vi "Redirect Assemblies in Veristand Steps Project XML.vi"() -> ()   [LabVIEW 2013, in "Assembly Redirection VIs.lvlib"]
uses:
  Assembly Redirection VIs.lvlib
  <vilib>/xml/NI_XML.lvlib
  <resource>/objmgr/DOMUserDefRef.rc
  <vilib>/xml/Load XML File.vi
  <vilib>/xml/Close Reference(Node).vi
  <vilib>/ni/Simple XML/Simple XML.lvlib
  <vilib>/xml/Close Reference(NNMap).vi
  <vilib>/NI/Simple XML/_polymorphics/Create Tag - Child with Text.vi
panel:
  in  "New VS Assembly Version":string="2016.0.0.0"
  in  "New VS Assembly Version (GAC)":string="4.0.2016.0.9.9"
  out "New Assembly Reference Include Strings":string[](array[string])=["NationalInstruments.TestStand.Interop.API, Version=1.2.3.4, Culture=neutral, PublicKeyToken=ad9244eb3b825cd8, processorArchitecture=MSIL", "NationalInstruments.TestStand.Interop.UI, Version=1.2.3.4, Culture=neutral, PublicKeyToken=ad9244eb3b825cd8, processorArchitecture=MSIL", "NationalInstruments.TestStand.Interop.UI.AxControls, Version=1.2.3.4, Culture=neutral, PublicKeyToken=ad9244eb3b825cd8, processorArchitecture=MSIL", "NationalInstruments.TestStand.Interop.UI.Support, Version=1.2.3.4, Culture=neutral, PublicKeyToken=ad9244eb3b825cd8, processorArchitecture=MSIL", "NationalInstruments.TestStand.Interop.Utility, Version=5.6.7.8, Culture=neutral, processorArchitecture=x86", "NationalInstruments.VeriStand, Version=2016.0.0.0, Culture=neutral, PublicKeyToken=a6d690c380daa308, processorArchitecture=MSIL", "NationalInstruments.VeriStand.ClientAPI, Version=2016.0.0.0, Culture=neutral, PublicKeyToken=a6d690c380daa308, processorArchitecture=MSIL", "NationalInstruments.VeriStand.DataTypes, Version=2016.0.0.0, Culture=neutral, PublicKeyToken=a6d690c380daa308, processorArchitecture=MSIL", "NationalInstruments.VeriStand.RealTimeSequenceDefinitionApi, Version=2016.0.0.0, Culture=neutral, PublicKeyToken=a6d690c380daa308, processorArchitecture=MSIL", "NationalInstruments.VeriStand.SystemDefinitionAPI, Version=2016.0.0.0, Culture=neutral, PublicKeyToken=a6d690c380daa308, processorArchitecture=MSIL", "NationalInstruments.VeriStand.SystemStorage, Version=2016.0.0.0, Culture=neutral, PublicKeyToken=a6d690c380daa308, processorArchitecture=MSIL", "NationalInstruments.VeriStand.SystemStorageUI, Version=2016.0.0.0, Culture=neutral, PublicKeyToken=a6d690c380daa308, processorArchitecture=MSIL", "NationalInstruments.VeriStand.WorkspaceMacro, Version=2016.0.0.0, Culture=neutral, PublicKeyToken=a6d690c380daa308, processorArchitecture=MSIL"]
  out "New Assembly HintPath Properties":string[](array[string])=["..\\..\\..\\..\\..\\..\\..\\..\\..\\Program Files (x86)\\National Instruments\\TestStand 2016\\API\\DotNet\\Assemblies\\CurrentVersion\\NationalInstruments.TestStand.Interop.API.dll", "..\\..\\..\\..\\..\\..\\..\\..\\..\\Program Files (x86)\\National Instruments\\TestStand 2016\\API\\DotNet\\Assemblies\\CurrentVersion\\NationalInstruments.TestStand.Interop.UI.dll", "..\\..\\..\\..\\..\\..\\..\\..\\..\\Program Files (x86)\\National Instruments\\TestStand 2016\\API\\DotNet\\Assemblies\\CurrentVersion\\NationalInstruments.TestStand.Interop.UI.AxControls.dll", "..\\..\\..\\..\\..\\..\\..\\..\\..\\Program Files (x86)\\National Instruments\\TestStand 2016\\API\\DotNet\\Assemblies\\CurrentVersion\\NationalInstruments.TestStand.Interop.UISupport.dll", "..\\..\\..\\..\\..\\..\\..\\..\\..\\Program Files (x86)\\National Instruments\\TestStand 2016\\Bin\\NationalInstruments.TestStand.Utility.dll", "..\\..\\..\\..\\..\\..\\..\\..\\Windows\\Microsoft.NET\\assembly\\GAC_MSIL\\NationalInstruments.VeriStand\\v4.0_2016.0.9.9__a6d690c380daa308\\NationalInstruments.VeriStand.dll", "..\\..\\..\\..\\..\\..\\..\\..\\Windows\\Microsoft.NET\\assembly\\GAC_MSIL\\NationalInstruments.VeriStand.ClientAPI\\v4.0_2016.0.9.9__a6d690c380daa308\\NationalInstruments.VeriStand.ClientAPI.dll", "..\\..\\..\\..\\..\\..\\..\\..\\Windows\\Microsoft.NET\\assembly\\GAC_MSIL\\NationalInstruments.VeriStand.DataTypes\\v4.0_2016.0.9.9__a6d690c380daa308\\NationalInstruments.VeriStand.DataTypes.dll", "..\\..\\..\\..\\..\\..\\..\\..\\Windows\\Microsoft.NET\\assembly\\GAC_MSIL\\NationalInstruments.VeriStand.RealTimeSequenceDefinitionAPI\\v4.0_2016.0.9.9__a6d690c380daa308\\NationalInstruments.VeriStand.RealTimeSequenceDefinitionAPI.dll", "..\\..\\..\\..\\..\\..\\..\\..\\Windows\\Microsoft.NET\\assembly\\GAC_MSIL\\NationalInstruments.VeriStand.SystemDefinitionAPI\\v4.0_2016.0.9.9__a6d690c380daa308\\NationalInstruments.VeriStand.SystemDefinition.dll", "..\\..\\..\\..\\..\\..\\..\\..\\Windows\\Microsoft.NET\\assembly\\GAC_MSIL\\NationalInstruments.VeriStand.SystemStorage\\v4.0_2016.0.9.9__a6d690c380daa308\\NationalInstruments.VeriStand.SystemStorage.dll", "..\\..\\..\\..\\..\\..\\..\\..\\Windows\\Microsoft.NET\\assembly\\GAC_MSIL\\NationalInstruments.VeriStand.SystemStorageUI\\v4.0_2016.0.9.9__a6d690c380daa308\\NationalInstruments.VeriStand.SystemStorageUI.dll", "..\\..\\..\\..\\..\\..\\..\\..\\Windows\\Microsoft.NET\\assembly\\GAC_MSIL\\NationalInstruments.VeriStand.WorkspaceMacro\\v4.0_2016.0.9.9__a6d690c380daa308\\NationalInstruments.VeriStand.WorkspaceMacro.dll"]
  in  "New TS Version":dbl=2016.0 format="%#_6f"
  out "error out":errorcluster
  in  "Path to New XML File":path=path "C:/Users/achurch/Documents/Source/XML Mutation Code/Examples XML Files/VeristandSteps_mod.csproj" caption="Path to New RemoveOldInsertionPaletteItems project file"
  in  "New TS Utility Assembly Version":string="5.6.7.8"
  in  "New TS Interop Assembly Version":string="1.2.3.4"
  in  "XML file path":path=path "C:/Users/achurch/Documents/Source/XML Mutation Code/Examples XML Files/VeristandSteps.csproj" caption="Path to Old RemoveOldInsertionPaletteItems project file"
  # "Arguments\n1: original path (string)\n2: new path (string)\n3: TS Version (2014)\n4: TS Interop Assembly Version (14.0.0.0)\n5: TS Utility Assembly Version (14.0.0.0)\n6: VS Assembly Version (GAC format, 4.0.2016.0.0.0)\n7: VS Assembly Version (2016.0.0.0)"
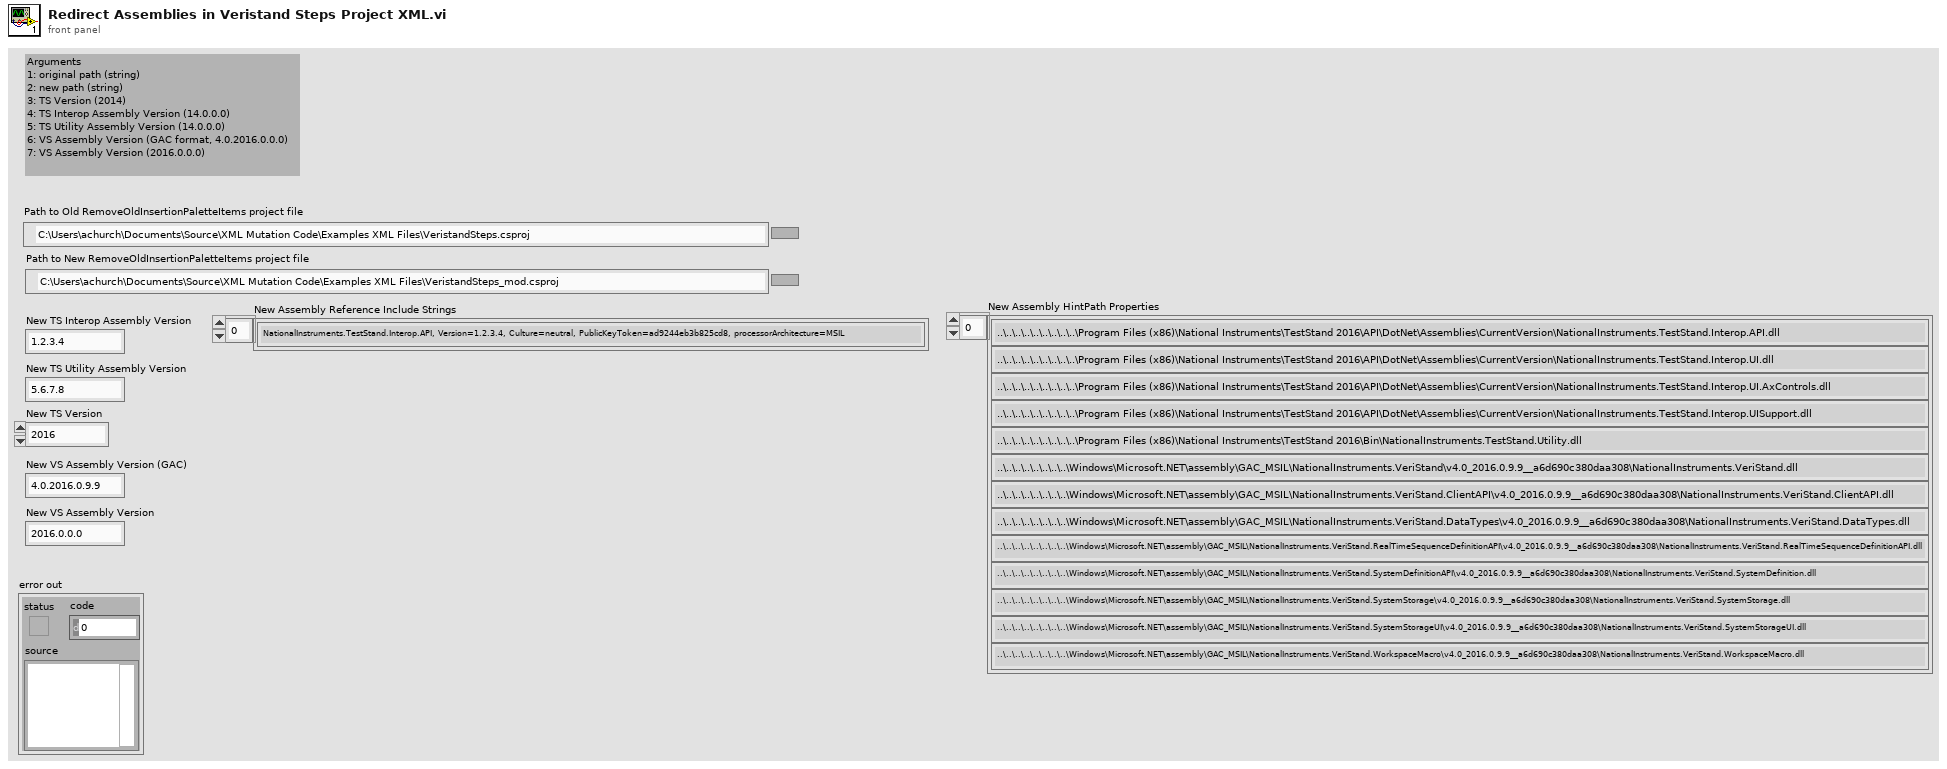
[diagram p1: front panel]
types:
  T1 = enum32{"invalid app kind", "Development System", "Run Time System", "Student Edition", "Embedded LabVIEW", "Evaluation", "Custom"}
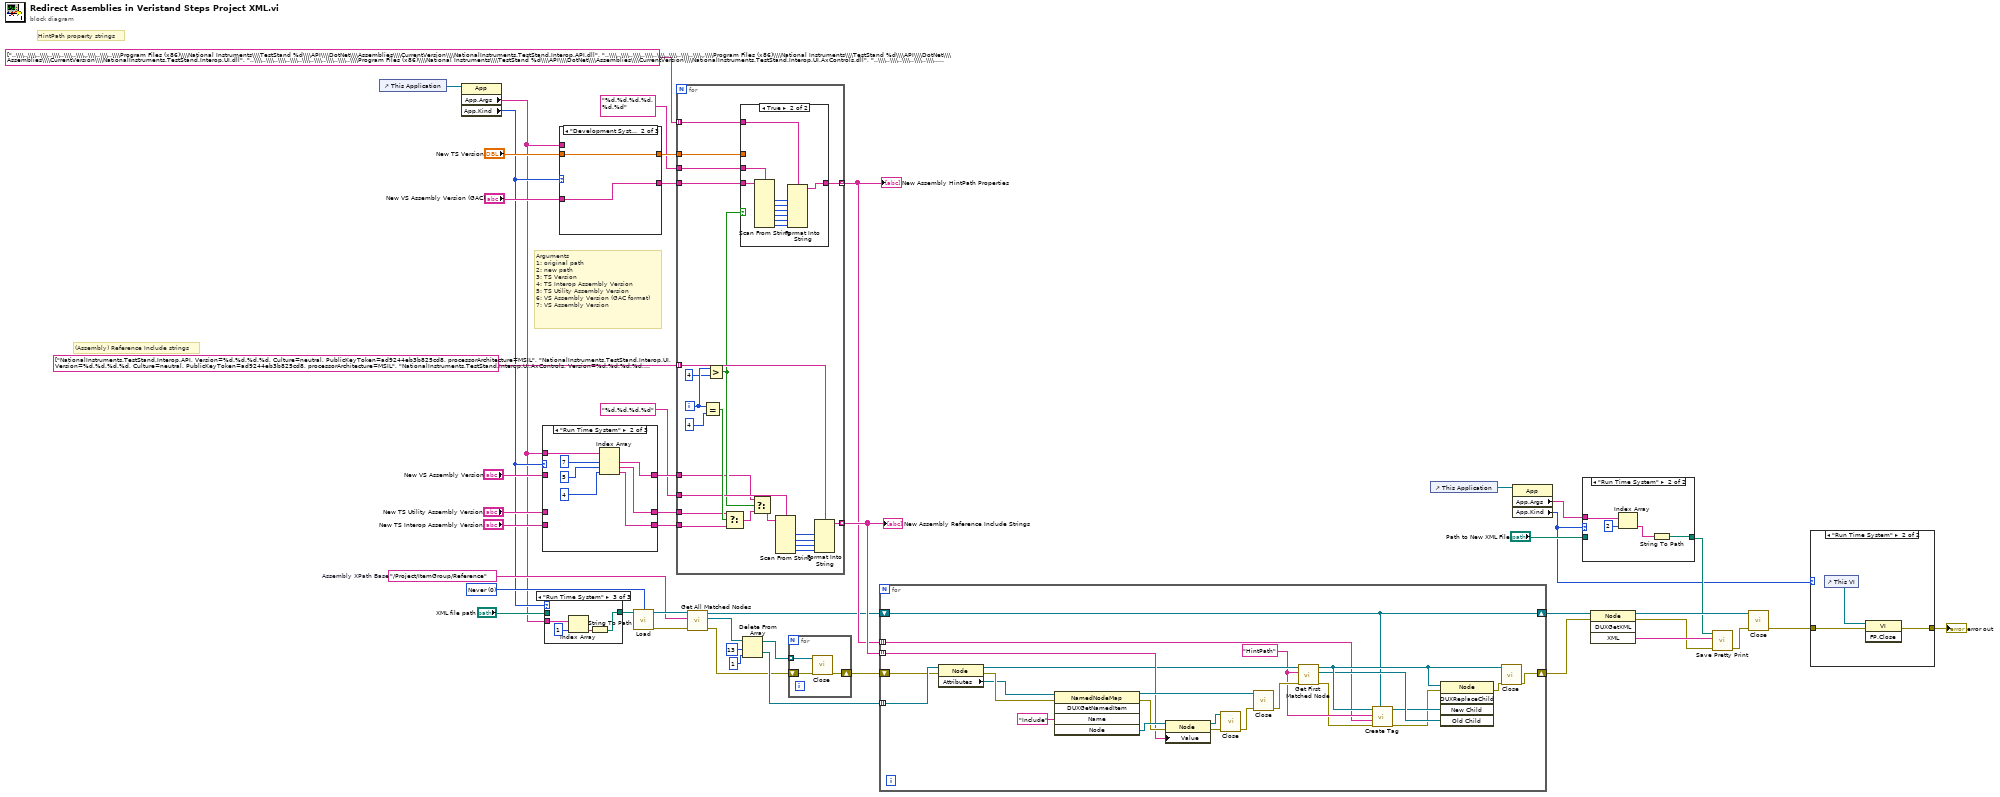
[diagram p0: block diagram]
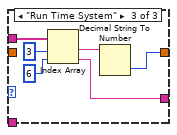
[diagram p9: hidden frame]
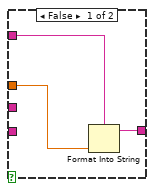
[diagram p10: hidden frame]
diagram:
  w43 = "/Project/ItemGroup/Reference"  # Assembly XPath Base
  w46 = 0 items=["Never", "Always", "Auto"] ("validate on load (Auto)")
  # "Arguments\n1: original path\n2: new path\n3: TS Version\n4: TS Interop Assembly Version\n5: TS Utility Assembly Version\n6: VS Assembly Version (GAC format)\n7: VS Assembly Version"
  # "(Assembly) Reference Include strings"
  # "HintPath property strings"
  n1 = control-ref of="This Application"() -> (w24:refnum<vi>)
  n2 = property class="App"(reference=w24) -> ("App.Args"=w8:string[], "App.Kind"=w11:T1)  [unwired: 1 in, 2 out]
  n3 = case shown="\"Run Time System\"" w11 {
    tunnel: [w49 w54 w59] -> w17
    tunnel: "New VS Assembly Version" -> [w49 _ w59]
    tunnel: [w48 w51 w58] -> w15
    tunnel: "New TS Utility Assembly Version" -> [w48 _ w58]
    tunnel: [w47 w50 w57] -> w13
    tunnel: "New TS Interop Assembly Version" -> [w47 _ w57]
    tunnel: w8 -> [_ w56 _]
    frame "Development System" {
    }
    frame "Run Time System" {
      n4 = Index Array(array=w56, index #1=7 ("index"), index #2=5 ("index"), index #3=4 ("index")) -> (element #1=w54:string, element #2=w51:string, element #3=w50:string)
    }
    frame Default {
    }
  }
  n5 = case shown="\"Run Time System\"" w11 {
    tunnel: "XML file path" -> [w60 w61 _]
    tunnel: [w60 w61 w63] -> w9
    tunnel: w8 -> [_ _ w64]
    frame "Development System" {
    }
    frame Default {
    }
    frame "Run Time System" {
      n6 = Index Array(array=w64, index=1) -> (element=w65:string)
      n7 = String To Path(string=w65) -> (path=w63:path)
    }
  }
  n8 = case shown="\"Development System\"" w11 {
    tunnel: "New TS Version" -> [_ w67 _]
    tunnel: "New VS Assembly Version (GAC)" -> [_ w66 _]
    tunnel: [_ w67 w69] -> w21
    tunnel: [_ w66 w68] -> w20
    tunnel: w8 -> [_ _ w73]
    frame Default {
    }
    frame "Development System" {
    }
    frame "Run Time System" {
      n9 = Index Array(array=w73, index #1=3 ("index"), index #2=6 ("index")) -> (element #1=w70:string, element #2=w68:string)
      n10 = Decimal String To Number(string=w70) -> (number=w69:i32)  [unwired: 2 in, 1 out]
    }
  }
  n11 = call-poly <vilib>:"Load.vi"("path to XML document"=w9, "validate on load (Auto)"=w46) -> ("DOM document out"=w44:refnum<k20>, "error out"=w45:errorcluster)  [unwired: 11 in, 1 out]
  n12 = for {
    tunnel: w15 -> [w93]
    tunnel: w13 -> [w94]
    tunnel: "%d.%d.%d.%d" ("format string") -> [w92]
    tunnel: string[] ["NationalInstruments.TestStand.Interop.API, Version=%d.%d.%d.%d, Culture=neutral, PublicKeyToken=ad9244eb3b825cd8, processorArchitecture=MSIL", "NationalInstruments.TestStand.Interop.UI, Version=%d.%d.%d.%d, Culture=neutral, PublicKeyToken=ad9244eb3b825cd8, processorArchitecture=MSIL", "NationalInstruments.TestStand.Interop.UI.AxControls, Version=%d.%d.%d.%d, Culture=neutral, PublicKeyToken=ad9244eb3b825cd8, processorArchitecture=MSIL", "NationalInstruments.TestStand.Interop.UI.Support, Version=%d.%d.%d.%d, Culture=neutral, PublicKeyToken=ad9244eb3b825cd8, processorArchitecture=MSIL", "NationalInstruments.TestStand.Interop.Utility, Version=%d.%d.%d.%d, Culture=neutral, processorArchitecture=x86", "NationalInstruments.VeriStand, Version=%d.%d.%d.%d, Culture=neutral, PublicKeyToken=a6d690c380daa308, processorArchitecture=MSIL", "NationalInstruments.VeriStand.ClientAPI, Version=%d.%d.%d.%d, Culture=neutral, PublicKeyToken=a6d690c380daa308, processorArchitecture=MSIL", "NationalInstruments.VeriStand.DataTypes, Version=%d.%d.%d.%d, Culture=neutral, PublicKeyToken=a6d690c380daa308, processorArchitecture=MSIL", "NationalInstruments.VeriStand.RealTimeSequenceDefinitionApi, Version=%d.%d.%d.%d, Culture=neutral, PublicKeyToken=a6d690c380daa308, processorArchitecture=MSIL", "NationalInstruments.VeriStand.SystemDefinitionAPI, Version=%d.%d.%d.%d, Culture=neutral, PublicKeyToken=a6d690c380daa308, processorArchitecture=MSIL", "NationalInstruments.VeriStand.SystemStorage, Version=%d.%d.%d.%d, Culture=neutral, PublicKeyToken=a6d690c380daa308, processorArchitecture=MSIL", "NationalInstruments.VeriStand.SystemStorageUI, Version=%d.%d.%d.%d, Culture=neutral, PublicKeyToken=a6d690c380daa308, processorArchitecture=MSIL", "NationalInstruments.VeriStand.WorkspaceMacro, Version=%d.%d.%d.%d, Culture=neutral, PublicKeyToken=a6d690c380daa308, processorArchitecture=MSIL"] -> [w91] mode=indexing
    tunnel: [w86] -> w34 mode=indexing
    tunnel: string[] ["..\\\\..\\\\..\\\\..\\\\..\\\\..\\\\..\\\\..\\\\..\\\\Program Files (x86)\\\\National Instruments\\\\TestStand %d\\\\API\\\\DotNet\\\\Assemblies\\\\CurrentVersion\\\\NationalInstruments.TestStand.Interop.API.dll", "..\\\\..\\\\..\\\\..\\\\..\\\\..\\\\..\\\\..\\\\..\\\\Program Files (x86)\\\\National Instruments\\\\TestStand %d\\\\API\\\\DotNet\\\\Assemblies\\\\CurrentVersion\\\\NationalInstruments.TestStand.Interop.UI.dll", "..\\\\..\\\\..\\\\..\\\\..\\\\..\\\\..\\\\..\\\\..\\\\Program Files (x86)\\\\National Instruments\\\\TestStand %d\\\\API\\\\DotNet\\\\Assemblies\\\\CurrentVersion\\\\NationalInstruments.TestStand.Interop.UI.AxControls.dll", "..\\\\..\\\\..\\\\..\\\\..\\\\..\\\\..\\\\..\\\\..\\\\Program Files (x86)\\\\National Instruments\\\\TestStand %d\\\\API\\\\DotNet\\\\Assemblies\\\\CurrentVersion\\\\NationalInstruments.TestStand.Interop.UISupport.dll", "..\\\\..\\\\..\\\\..\\\\..\\\\..\\\\..\\\\..\\\\..\\\\Program Files (x86)\\\\National Instruments\\\\TestStand %d\\\\Bin\\\\NationalInstruments.TestStand.Utility.dll", "..\\\\..\\\\..\\\\..\\\\..\\\\..\\\\..\\\\..\\\\Windows\\\\Microsoft.NET\\\\assembly\\\\GAC_MSIL\\\\NationalInstruments.VeriStand\\\\v%d.%d_%d.%d.%d.%d__a6d690c380daa308\\\\NationalInstruments.VeriStand.dll", "..\\\\..\\\\..\\\\..\\\\..\\\\..\\\\..\\\\..\\\\Windows\\\\Microsoft.NET\\\\assembly\\\\GAC_MSIL\\\\NationalInstruments.VeriStand.ClientAPI\\\\v%d.%d_%d.%d.%d.%d__a6d690c380daa308\\\\NationalInstruments.VeriStand.ClientAPI.dll", "..\\\\..\\\\..\\\\..\\\\..\\\\..\\\\..\\\\..\\\\Windows\\\\Microsoft.NET\\\\assembly\\\\GAC_MSIL\\\\NationalInstruments.VeriStand.DataTypes\\\\v%d.%d_%d.%d.%d.%d__a6d690c380daa308\\\\NationalInstruments.VeriStand.DataTypes.dll", "..\\\\..\\\\..\\\\..\\\\..\\\\..\\\\..\\\\..\\\\Windows\\\\Microsoft.NET\\\\assembly\\\\GAC_MSIL\\\\NationalInstruments.VeriStand.RealTimeSequenceDefinitionAPI\\\\v%d.%d_%d.%d.%d.%d__a6d690c380daa308\\\\NationalInstruments.VeriStand.RealTimeSequenceDefinitionAPI.dll", "..\\\\..\\\\..\\\\..\\\\..\\\\..\\\\..\\\\..\\\\Windows\\\\Microsoft.NET\\\\assembly\\\\GAC_MSIL\\\\NationalInstruments.VeriStand.SystemDefinitionAPI\\\\v%d.%d_%d.%d.%d.%d__a6d690c380daa308\\\\NationalInstruments.VeriStand.SystemDefinitionAPI.dll", "..\\\\..\\\\..\\\\..\\\\..\\\\..\\\\..\\\\..\\\\Windows\\\\Microsoft.NET\\\\assembly\\\\GAC_MSIL\\\\NationalInstruments.VeriStand.SystemStorage\\\\v%d.%d_%d.%d.%d.%d__a6d690c380daa308\\\\NationalInstruments.VeriStand.SystemStorage.dll", "..\\\\..\\\\..\\\\..\\\\..\\\\..\\\\..\\\\..\\\\Windows\\\\Microsoft.NET\\\\assembly\\\\GAC_MSIL\\\\NationalInstruments.VeriStand.SystemStorageUI\\\\v%d.%d_%d.%d.%d.%d__a6d690c380daa308\\\\NationalInstruments.VeriStand.SystemStorageUI.dll", "..\\\\..\\\\..\\\\..\\\\..\\\\..\\\\..\\\\..\\\\Windows\\\\Microsoft.NET\\\\assembly\\\\GAC_MSIL\\\\NationalInstruments.VeriStand.WorkspaceMacro\\\\v%d.%d_%d.%d.%d.%d__a6d690c380daa308\\\\NationalInstruments.VeriStand.WorkspaceMacro.dll"] -> [w85] mode=indexing
    tunnel: w21 -> [w78]
    tunnel: [w84] -> w27 mode=indexing
    tunnel: w20 -> [w80]
    tunnel: "%d.%d.%d.%d.%d.%d" ("format string") -> [w79]
    tunnel: w17 -> [w76]
    i -> [w82]
    n13 = Equal?(x=w82, y=4 ("x")) -> (x = y?=w95:bool)
    n14 = Greater?(x=w82, y=4 ("x")) -> (0:w77:bool)
    n15 = Select(t=w93, s=w95, f=w94) -> (s? t:f=w75:string)
    n16 = case shown="True" w77 {
      tunnel: w85 -> [w98 w108]
      tunnel: [w96 w107] -> w84
      tunnel: w80 -> [_ w106]
      tunnel: w79 -> [_ w105]
      tunnel: w78 -> [w97 _]
      frame False {
        n17 = Format Into String(format string=w98, w97) -> (resulting string=w96:string)  [unwired: 2 in, 1 out]
      }
      frame True {
        n18 = Scan From String(format string=w105, input string=w106) -> (output 1=w104:i32, output 2=w103:i32, output 3=w102:i32, output 4=w101:i32, output 5=w100:i32, output 6=w99:i32)  [unwired: 8 in, 3 out]
        n19 = Format Into String(format string=w108, w104, w103, w102, w101, w100, w99) -> (resulting string=w107:string)  [unwired: 2 in, 1 out]
      }
    }
    n20 = Select(t=w76, s=w77, f=w75) -> (s? t:f=w74:string)
    n21 = Scan From String(format string=w92, input string=w74) -> (output 1=w90:i32, output 2=w89:i32, output 3=w88:i32, output 4=w87:i32)  [unwired: 6 in, 3 out]
    n22 = Format Into String(format string=w91, w90, w89, w88, w87) -> (resulting string=w86:string)  [unwired: 2 in, 1 out]
  }
  "New Assembly HintPath Properties" <- w27
  "New Assembly Reference Include Strings" <- w34
  n23 = call <vilib>:"Get All Matched Nodes.vi"("error in (no error)"=w45, "XPath expression"=w43, "node in"=w44) -> ("error out"=w37:errorcluster, "node result array"=w42:refnum<k20>[], "node out"=w26:refnum<k20>)  [unwired: 6 in]
  n24 = Delete From Array(array=w42, length=13, index=1 ("length")) -> (deleted portion=w39:refnum<k20>[], array with subset deleted=w38:refnum<k20>[])
  n25 = for {
    tunnel: w38 -> [w111] mode=indexing
    shift-right: [w109] -> w36
    shift-left: w37 -> [w110]
    n26 = call-poly <vilib>:"Close.vi"("error in (no error)"=w110, "node"=w111) -> ("error out"=w109:errorcluster)  [unwired: 7 in]
  }
  n27 = for {
    tunnel: w39 -> [w132] mode=indexing
    shift-right: [w126] -> w33
    shift-left: w36 -> [w131]
    tunnel: w34 -> [w125] mode=indexing
    tunnel: w27 -> [w113] mode=indexing
    shift-right: [w112] -> w25
    shift-left: w26 -> [w112]
    w120 = "HintPath" ("XPath expression")
    n28 = property class="Node"(reference=w132, error in=w131) -> (reference out=w121:refnum<k20>, error out=w135:errorcluster, "Attributes"=w133:refnum<k20>)
    n29 = invoke class="NamedNodeMap" method="DUXGetNamedItem"(reference=w133, error in=w135, "Name"="Include") -> (reference out=w127:refnum<k20>, error out=w129:errorcluster, "Node"=w130:refnum<k20>)  [unwired: 2 in, 2 out]
    n30 = property class="Node"(reference=w130, error in=w129, "Value"=w125) -> (reference out=w128:refnum<k20>, error out=w124:errorcluster)
    n31 = call-poly <vilib>:"Close.vi"("error in (no error)"=w124, "node"=w128) -> ("error out"=w123:errorcluster)  [unwired: 7 in]
    n32 = call-poly <vilib>:"Close.vi"("error in (no error)"=w123, "named node map"=w127) -> ("error out"=w122:errorcluster)  [unwired: 7 in]
    n33 = call <vilib>:"Get First Matched Node.vi"("error in (no error)"=w122, "XPath expression"=w120, "node in"=w121) -> ("error out"=w119:errorcluster, "node result"=w117:refnum<k20>, "node out"=w118:refnum<k20>)  [unwired: 6 in]
    n34 = call-poly <vilib>:"Create Tag.vi"("DOM document reference"=w112, "error in (no error)"=w119, "Text Data"=w113, "Tag Name"=w120, "Parent Element reference"=w118) -> ("error out"=w115:errorcluster, "Child Element reference"=w116:refnum<k20>)  [unwired: 5 in]
    n35 = invoke class="Node" method="DUXReplaceChild"(reference=w118, error in=w115, "New Child"=w116, "Old Child"=w117) -> (error out=w114:errorcluster)  [unwired: 1 in, 4 out]
    n36 = call-poly <vilib>:"Close.vi"("error in (no error)"=w114, "node"=w118) -> ("error out"=w126:errorcluster)  [unwired: 7 in]
  }
  n37 = control-ref of="This Application"() -> (w6:refnum<vi>)
  n38 = property class="App"(reference=w6) -> ("App.Args"=w5:string[], "App.Kind"=w3:T1)  [unwired: 1 in, 2 out]
  n39 = case shown="\"Run Time System\"" w3 {
    tunnel: "Path to New XML File" -> [w136 _]
    tunnel: w5 -> [_ w140]
    tunnel: [w136 w137] -> w4
    frame "Development System", Default {
    }
    frame "Run Time System" {
      n40 = Index Array(array=w140, index=2) -> (element=w138:string)
      n41 = String To Path(string=w138) -> (path=w137:path)
    }
  }
  n42 = invoke class="Node" method="DUXGetXML"(reference=w25, error in=w33) -> (reference out=w29:refnum<k20>, error out=w31:errorcluster, "XML"=w32:string)  [unwired: 2 in, 1 out]
  n43 = call <vilib>:"Save Pretty Print.vi"("error in (no error)"=w31, "Pretty XML String"=w32, "XML file path"=w4) -> ("error out"=w30:errorcluster)  [unwired: 7 in, 1 out]
  n44 = call-poly <vilib>:"Close.vi"("error in (no error)"=w30, "node"=w29) -> ("error out"=w2:errorcluster)  [unwired: 7 in]
  n45 = case shown="\"Run Time System\"" w3 {
    tunnel: w2 -> [w141 w143]
    tunnel: [w141 w142] -> w1
    frame "Development System", Default {
    }
    frame "Run Time System" {
      n46 = control-ref of="This VI"() -> (w144:refnum<vi>)
      n47 = invoke class="VI" method="FP.Close"(reference=w144, error in=w143) -> (error out=w142:errorcluster)  [unwired: 1 in, 2 out]
    }
  }
  "error out" <- w1
